vi "GetI.vi"(8 "error in (no error)":errorcluster, 11 "reference in":refnum<class "GOOP4_Base.lvclass">) -> (0 "error out":errorcluster, 2 "i":i32, 3 "reference out":refnum<class "GOOP4_Base.lvclass">)   [LabVIEW 2019, in "GOOP4_Base.lvclass"]
uses:
  GOOP4_Base.lvclass
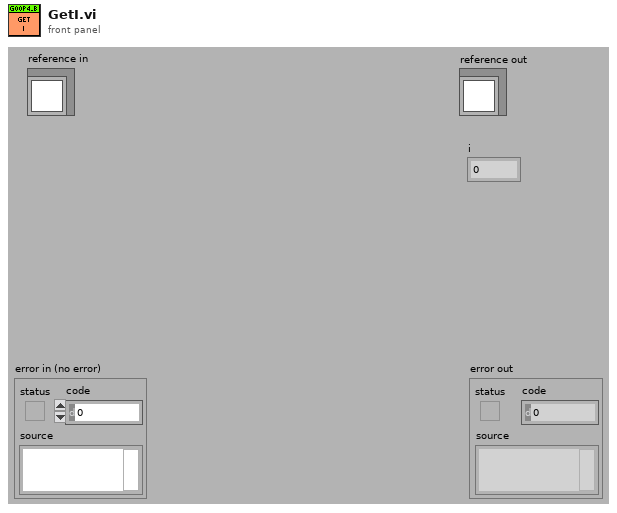
[diagram p1: front panel]
types:
  T1 = typedef "GOOP4_Base.lvclass/ObjectAttributes.ctl" = cluster{"i":i32}
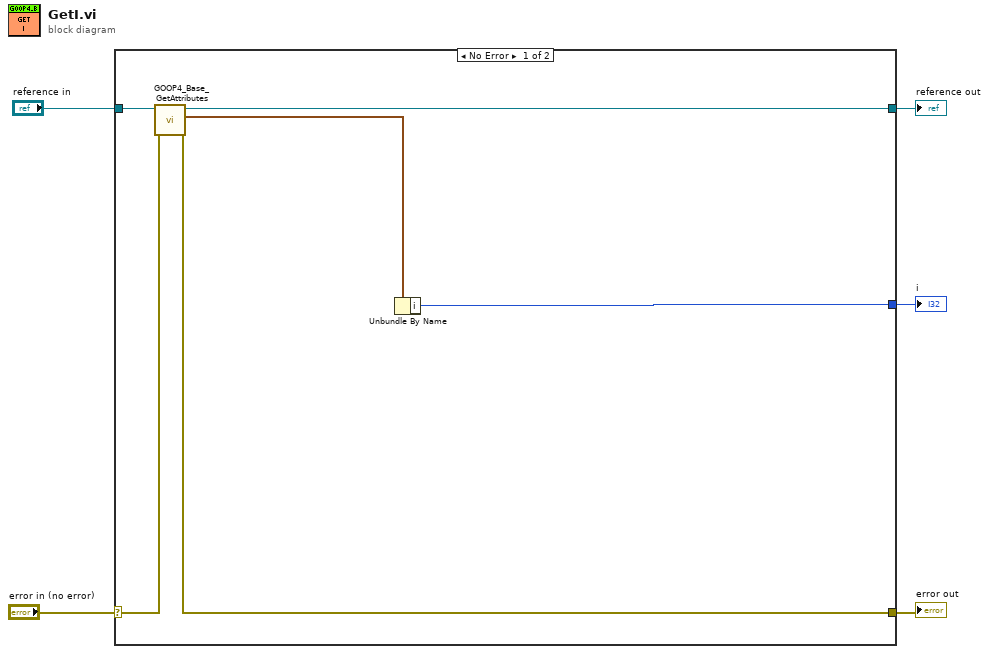
[diagram p0: block diagram]
diagram:
  n1 = case shown="No Error" "error in (no error)" {
    selector: "error in (no error)" -> [w11 w13]
    tunnel: [w9 w13] -> w4
    tunnel: [w7 w12] -> w2
    tunnel: "reference in" -> [w8 w12]
    tunnel: [w6 _] -> w1
    frame No Error {
      n2 = call "GOOP4_Base_GetAttributes.vi"("error in (no error)"=w11, "reference in"=w8) -> ("error out"=w9:errorcluster, "Data"=w10:T1, "reference out"=w7:refnum<class "GOOP4_Base.lvclass">)  [unwired: 6 in, 1 out]
      n3 = Unbundle By Name(w10) -> ("i"=w6:i32)
    }
    frame Error {
    }
  }
  "error out" <- w4
  "reference out" <- w2
  "i" <- w1
